vi "_tmp.vi"() -> ()   [LabVIEW 2019]
uses:
  lib/Element.ctl
  lib/Element Type.ctl
  lib/labview_json.lvlib
panel:
  in  "Cluster":cluster{"c":bool}
  out "JSON":string
  out "Exists? 2":bool
  in  "JSON Path":string[](array[string])=["c"]
  out "Exists?":bool
  out "error out":errorcluster
  out "Value":T1
  out "Keys/Indexes":string[](array[string])
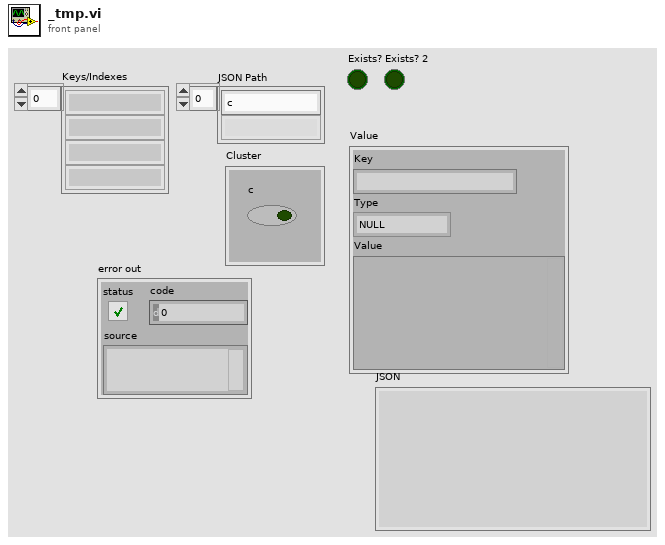
[diagram p1: front panel]
types:
  T1 = typedef "labview_json.lvlib/Element.ctl" = cluster{"Key":string, "Type":T2, "Value":variant}
  T2 = typedef "labview_json.lvlib/Element Type.ctl" = enum8{"NULL", "OBJECT", "ARRAY", "BOOL", "INT", "UINT", "FLOAT", "STRING"}
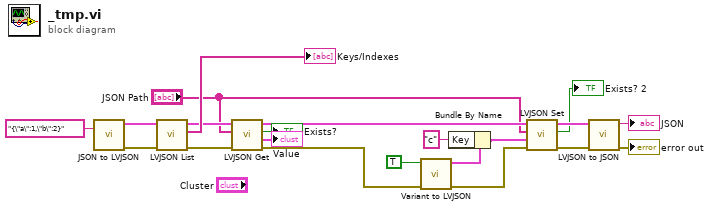
[diagram p0: block diagram]
diagram:
  n1 = call "JSON to LVJSON.vi"("JSON in"="{\"a\":1,\"b\":2}" ("JSON")) -> ("error out"=w19:errorcluster, "Root Element out"=w20:T1)  [unwired: 9 in]
  n2 = call "LVJSON List.vi"("error in (no error)"=w19, "Root Element in"=w20) -> ("error out"=w9:errorcluster, "Keys/Indexes"=→"Keys/Indexes":string[], "dup Root Element"=w17:T1)  [unwired: 6 in, 1 out]
  n3 = call "LVJSON Get.vi"("error in (no error)"=w9, "Root Path"="JSON Path", "Root Element in"=w17) -> ("error out"=w8:errorcluster, "Element out"=→"Value":T1, "Exists?"=→"Exists?":bool, "dup Root Element"=w16:T1)  [unwired: 5 in]
  n4 = call "Variant to LVJSON.vi"("error in (no error)"=w8, "Variant in"=TRUE) -> ("error out"=w7:errorcluster, "Element out"=w6:T1)  [unwired: 8 in]
  n5 = Bundle By Name(cluster=w6, "Key"="c") -> (w2:T1)
  n6 = call "LVJSON Set.vi"("error in (no error)"=w7, "Element"=w2, "Root Path"="JSON Path", "Root Element in"=w16) -> ("error out"=w15:errorcluster, "Exists?"=→"Exists? 2":bool, "Root Element out"=w14:T1)  [unwired: 5 in]
  n7 = call "LVJSON to JSON.vi"("error in (no error)"=w15, "Root Element in"=w14) -> ("error out"=→"error out":errorcluster, "JSON out"=→"JSON":string)  [unwired: 7 in, 1 out]
